vi "Open JSON Config File.vi"(8 "error in (no error)":errorcluster, 11 "Path":path) -> (0 "error out":errorcluster, 3 "JSON Config File out":refnum<class "JSON Config File.lvclass">)   [LabVIEW 2013, in "JSON Config File.lvclass"]
uses:
  JSON Config File.lvclass
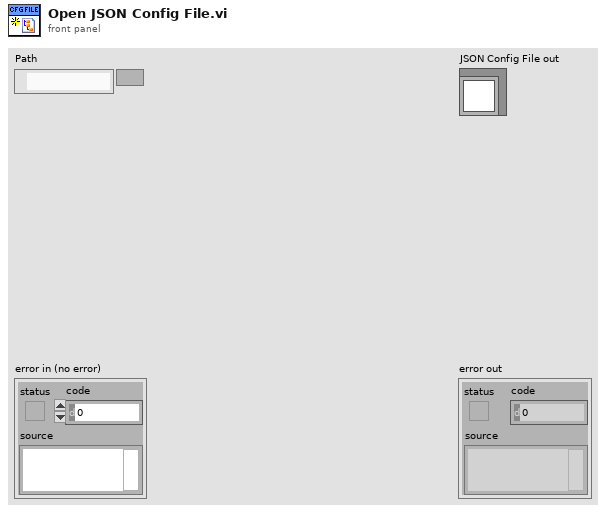
[diagram p1: front panel]
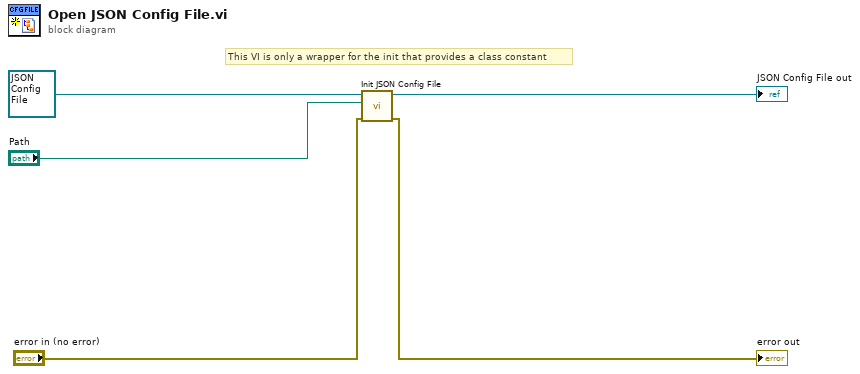
[diagram p0: block diagram]
diagram:
  # "This VI is only a wrapper for the init that provides a class constant"
  n1 = call "Init JSON Config File.vi"("error in (no error)"="error in (no error)", "Path"="Path", "JSON Config File in"=refnum<class "JSON Config File.lvclass"> refnum) -> ("error out"=→"error out":errorcluster, "JSON Config File out"=→"JSON Config File out":refnum<class "JSON Config File.lvclass">)  [unwired: 7 in]
